vi "uart.vi"() -> ()   [LabVIEW 2017]
uses:
  <vilib>/Instr/_visa.llb/VISA Configure Serial Port (Instr).vi
panel:
  in  "VISA resource name":refnum<visa-resource-name>
  out "error out":errorcluster
  in  "stop":bool
  in  "OK Button":bool
  out "read buffer":string
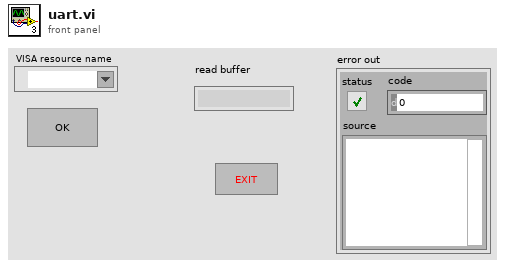
[diagram p1: front panel]
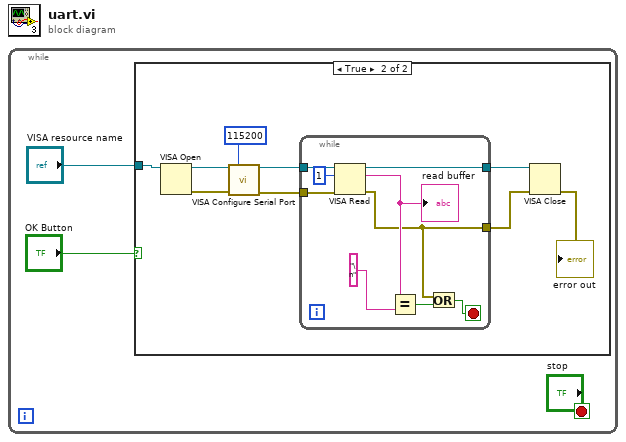
[diagram p0: block diagram]
diagram:
  n1 = while {
    stop <- "stop" stop-if-true
    n2 = case shown="True" "OK Button" {
      tunnel: "VISA resource name" -> [_ w9]
      frame False {
      }
      frame True {
        n3 = VISA Open(VISA resource name=w9) -> (VISA resource name=w8:refnum<visa-resource-name>, error out=w7:errorcluster)  [unwired: 4 in]
        n4 = call-poly "VISA Configure Serial Port"("VISA resource name"=w8, "baud rate (9600)"=u32 115200, "error in (no error)"=w7) -> ("VISA resource name out"=w5:refnum<visa-resource-name>, "error out"=w6:errorcluster)  [unwired: 11 in]
        n5 = while {
          tunnel: [w21] -> w12
          tunnel: w6 -> [w18]
          tunnel: [w15] -> w11
          tunnel: w5 -> [w13]
          stop <- w17 stop-if-true
          n6 = VISA Read(VISA resource name=w13, byte count=u32 1, error in (no error)=w18) -> (VISA resource name out=w21:refnum<visa-resource-name>, read buffer=w20:string, error out=w15:errorcluster)  [unwired: 1 out]
          "read buffer" <- w20
          n7 = Equal?(x=w20, y="\n") -> (x = y?=w16:bool)
          n8 = Or(x=w15, y=w16) -> (x .or. y?=w17:bool)
        }
        n9 = VISA Close(VISA resource name=w12, error in (no error)=w11) -> (error out=→"error out":errorcluster)
      }
    }
  }
